vi "Load PQ .bin Data.vi"(4 "# Pixels Y":i32, 6 "# Pixels X":i32, 8 "error in (no error)":errorcluster, 9 "# TCSPC Bins":i32, 10 "offset":i64, 11 "path in":path) -> (0 "error out":errorcluster, 2 "Array":i32[][][](array[numeric]), 3 "path out":path)   [LabVIEW 2021, in "PicoQuant.lvlib"]
uses:
  PicoQuant.lvlib
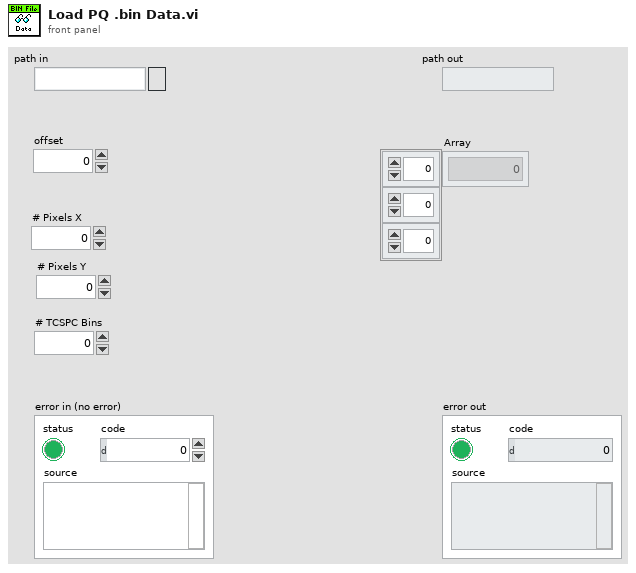
[diagram p1: front panel]
types:
  T1 = enum16{"big-endian, network order", "native, host order", "little-endian"}
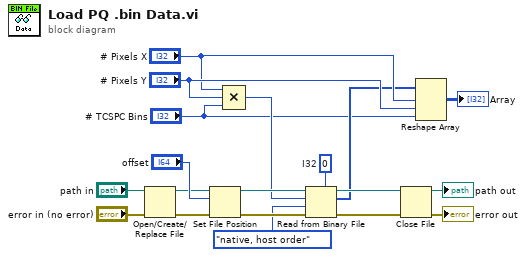
[diagram p0: block diagram]
diagram:
  w7 = 0  # I32
  n1 = Open/Create/Replace File(file path (use dialog)="path in", error in="error in (no error)") -> (refnum out=w13:refnum<file>, error out=w14:errorcluster)  [unwired: 4 in, 1 out]
  n2 = Set File Position(offset (in bytes) (0)="offset", refnum=w13, error in=w14) -> (refnum out=w17:refnum<file>, error out=w16:errorcluster)  [unwired: 1 in]
  n3 = Compound Arithmetic op=MULTIPLY("# Pixels X", "# Pixels Y", "# TCSPC Bins") -> (w4:i32)
  n4 = Read from Binary File(5:w7, 8:w16, 9:T1."native, host order" ("byte order (0:big-endian, network order)"), 10:w4, 11:w17) -> (0:w2:errorcluster, 2:w5:i32[], 3:w18:refnum<file>)  [unwired: 1 in, 1 out]
  n5 = Close File(refnum=w18, error in=w2) -> (path=→"path out":path, error out=→"error out":errorcluster)
  n6 = Reshape Array(w5, "# Pixels X", "# Pixels Y", "# TCSPC Bins") -> (→"Array":i32[][][])
